vi "G.vi"(9 "Z":u32 format="%08x", 10 "Y":u32 format="%08x", 11 "X":u32 format="%08x") -> (3 "G":u32 format="%08x")   [LabVIEW 2013, in "MD5.lvlib" / "MD5.lvclass"]
uses:
  MD5.lvclass
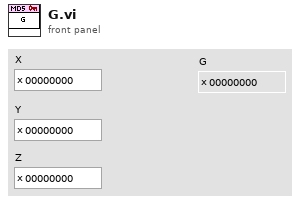
[diagram p1: front panel]
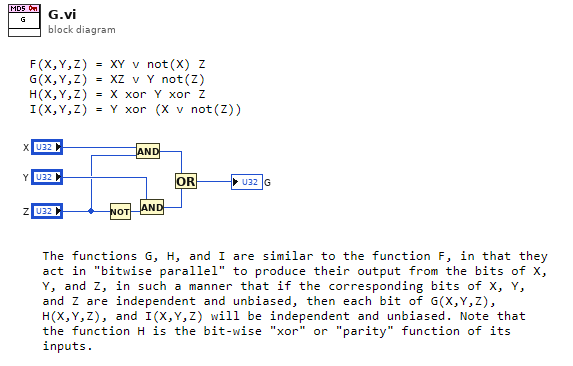
[diagram p0: block diagram]
diagram:
  n1 = Not(x="Z") -> (.not. x?=w1:u32)
  n2 = And(x="X", y="Z") -> (x .and. y?=w6:u32)
  n3 = And(x="Y", y=w1) -> (x .and. y?=w5:u32)
  n4 = Or(x=w6, y=w5) -> (x .or. y?=→"G":u32)
